vi "Decode Inverter Enable States.vi"(11 "Numeric":u8) -> (3 "Inv. Enable":enum16{"Inverter Disabled", "Inverter Enabled"}(ring))   [LabVIEW 2014]
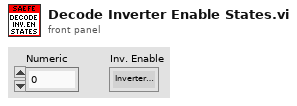
[diagram p1: front panel]
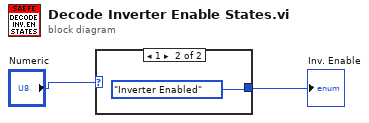
[diagram p0: block diagram]
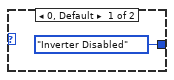
[diagram p2: hidden frame]
diagram:
  n1 = case shown="1" "Numeric" {
    tunnel: [enum16{"Inverter Disabled", "Inverter Enabled"}."Inverter Disabled" ("Inv. Enable") enum16{"Inverter Disabled", "Inverter Enabled"}."Inverter Enabled" ("Inv. Enable")] -> w2
    frame 0, Default {
    }
    frame 1 {
    }
  }
  "Inv. Enable" <- w2
